vi "Ask_561_power.vi"(8 "error in":errorcluster, 11 "VISA resource name":refnum<visa-resource-name>) -> (0 "error out":errorcluster, 2 "561 Power":dbl, 3 "VISA resource name out":refnum<visa-resource-name>)   [LabVIEW 2015]
panel:
  out "Serial Settings:Number of Bytes at Serial Port":u32
  out "read buffer":string
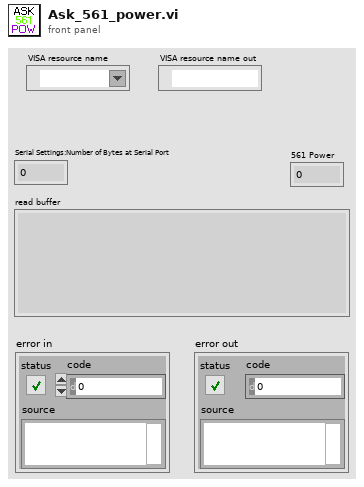
[diagram p1: front panel]
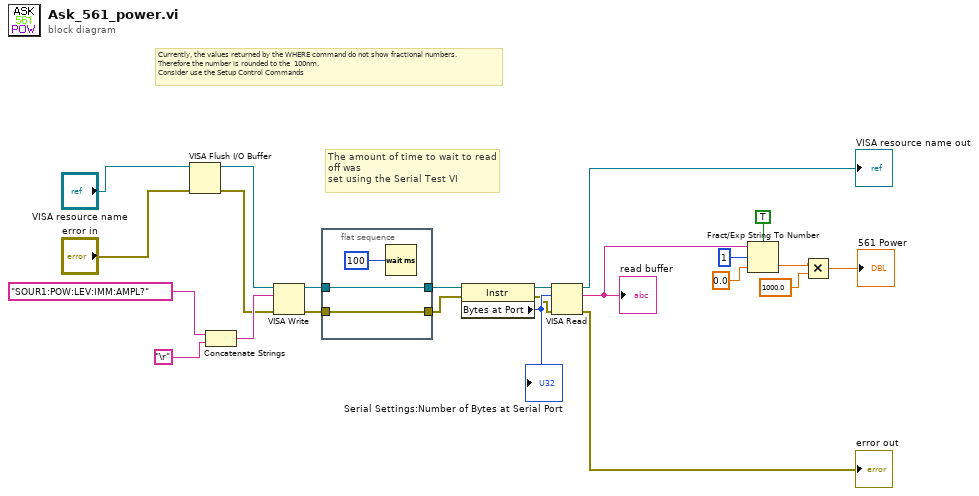
[diagram p0: block diagram]
diagram:
  # "Currently, the values returned by the WHERE command do not show fractional numbers.\nTherefore the number is rounded to the  100nm. \nConsider use the Setup Control Commands"
  # "The amount of time to wait to read off was \nset using the Serial Test VI"
  n1 = VISA Flush I/O Buffer(VISA resource name="VISA resource name", error in (no error)="error in") -> (VISA resource name out=w1:refnum<visa-resource-name>, error out=w3:errorcluster)  [unwired: 1 in]
  n2 = Concatenate Strings("SOUR1:POW:LEV:IMM:AMPL?" ("string"), "\r") -> (w14:string)
  n3 = VISA Write(VISA resource name=w1, write buffer=w14, error in (no error)=w3) -> (VISA resource name out=w20:refnum<visa-resource-name>, error out=w18:errorcluster)  [unwired: 1 out]
  n4 = flat-sequence {
    tunnel: [w26] -> w21
    tunnel: w20 -> [w26]
    tunnel: [w24] -> w19
    tunnel: w18 -> [w24]
    frame #0 {
      n5 = Wait (ms)(milliseconds to wait=u32 100) -> ()  [unwired: 1 out]
    }
  }
  n6 = property class="Instr"(reference=w21, error in=w19) -> (reference out=w23:refnum<visa-resource-name>, error out=w17:errorcluster, "Bytes at Port"=w22:u32)
  "Serial Settings:Number of Bytes at Serial Port" <- w22
  n7 = VISA Read(VISA resource name=w23, byte count=w22, error in (no error)=w17) -> (VISA resource name out=→"VISA resource name out":refnum<visa-resource-name>, read buffer=w6:string, error out=→"error out":errorcluster)  [unwired: 1 out]
  "read buffer" <- w6
  n8 = Fract/Exp String To Number(use system decimal point (T)=TRUE, string=w6, offset=1, default (0 dbl)=0.0 ("default (0 I32)")) -> (number=w8:dbl)  [unwired: 1 out]
  n9 = Multiply(x=w8, y=1000.0) -> (x*y=→"561 Power":dbl)
